vi "Manual Assembly DB_Nov2024.vi"() -> ()   [LabVIEW 2021]
uses:
  Classes/Assembly/Assembly Run.lvclass
  Classes/Workspace/Fixture Enum.ctl
  Classes/Workspace/Fixture.lvclass
  Classes/Controller/Controller.lvclass
  Classes/Assembly/Database Entry/Database Entry.lvclass
  SubVIs/component_tray_region.vi
  SubVIs/assembly_tray_region.vi
  SubVIs/PUT_region.vi
  <vilib>/JDP Science/JDP Science Common Utilities/JDP Utility.lvlib
  <vilib>/Utility/file.llb/Read Delimited Spreadsheet (string).vi
  Classes/Routine/Routine Enum.ctl
  Classes/Routine/Routine.lvclass
panel:
  out "Feet check":bool
  in  "Pick and Place 3":bool
  in  "Pick and Place 2":bool
  out "Assembly Type":string[](array[string])
  out "Assembly tray region":dbl
  out "Component tray region":dbl
  out "PUT Region":dbl
  in  "Clear All":bool
  in  "Assemble":bool
  in  "Pick and Place":bool
  in  "Dispense glue":bool
  in  "Go":bool
  in  "Routine":T1=enum."Dispense Epoxy"
  in  "Update":bool
  in  "Stage":i32(listbox)=-1
  in  "Stop":bool
  in  "Remove":bool
  in  "Add":bool
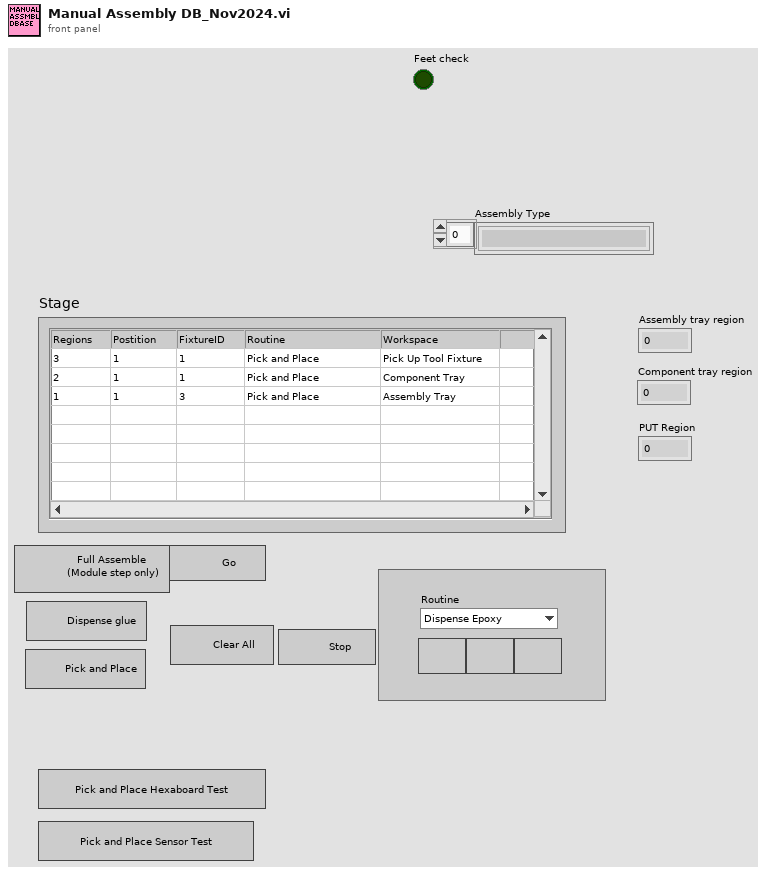
[diagram p1: front panel]
types:
  T1 = typedef "Routine.lvclass/Routine Enum.ctl" = enum16{"Primary Pick Up", "Secondary Pick Up", "Put Down All", "Secure Syringe", "Release Syringe", "Dispense Epoxy", "Pick Up All", "Put Down Secondary", "Full Assembly"}
  T2 = typedef "Fixture.lvclass/Fixture Enum.ctl" = enum16{"Assembly Tray", "Syringe Space", "Component", "Pick Up Tool", "Current Position"}
  T3 = typedef "File Paths.ctl" = cluster{"Glue Pattern Folder":path, "Carrier Tray Folder":path, "Pick Up Tool Fixture Folder":path, "Components Folder":path, "Bellows Tool Offset.txt":path, "Pick Up Tool Offset.txt":path, "Dispense Tip Offset.txt":path, "Log Files":path, "Gantry Assembly Map.txt":path, "Syringe and offset map.txt":path, "Controllers Folder":path, "Local dbase config":path}
  T4 = cluster{"Fixture ID":dbl, "Position":dbl, "Thickness":dbl}[]
  T5 = cluster{"Fixture ID":dbl, "Position":dbl, "Thickness":dbl}
  T6 = typedef "Controller.lvclass/Controllers.ctl" = cluster{"I-O.lvclass":refnum<class "I-O.lvclass">, "Gantry":refnum<k24>, "Dispenser":refnum<visa-resource-name>}
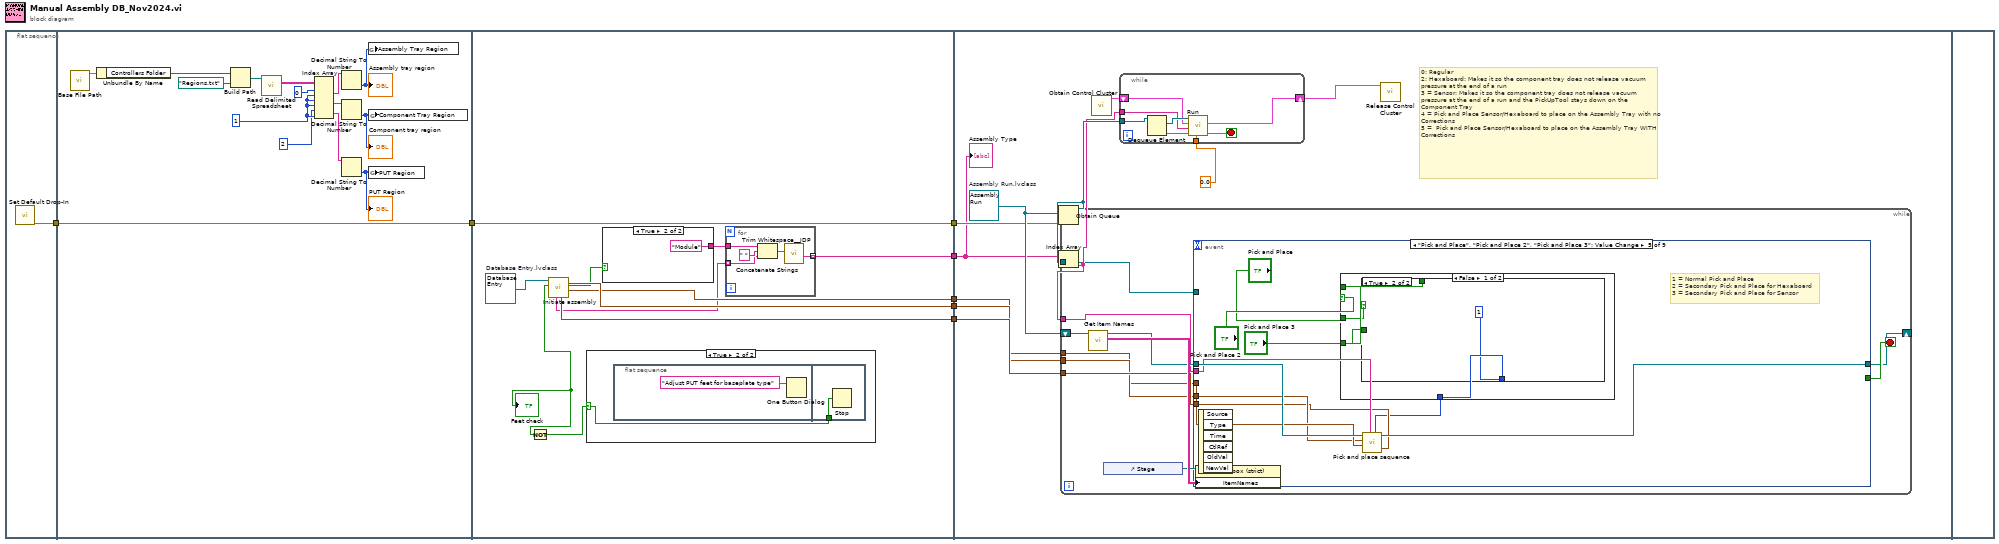
[diagram p0: block diagram]
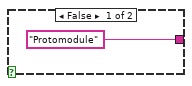
[diagram p3: hidden frame]
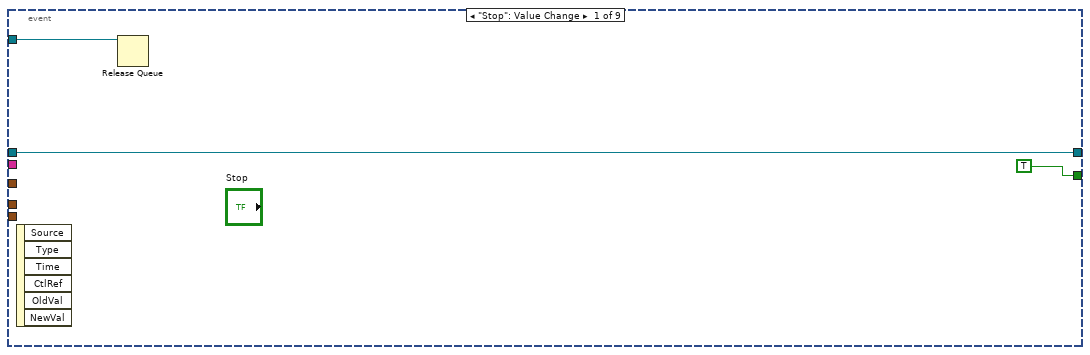
[diagram p4: hidden frame]
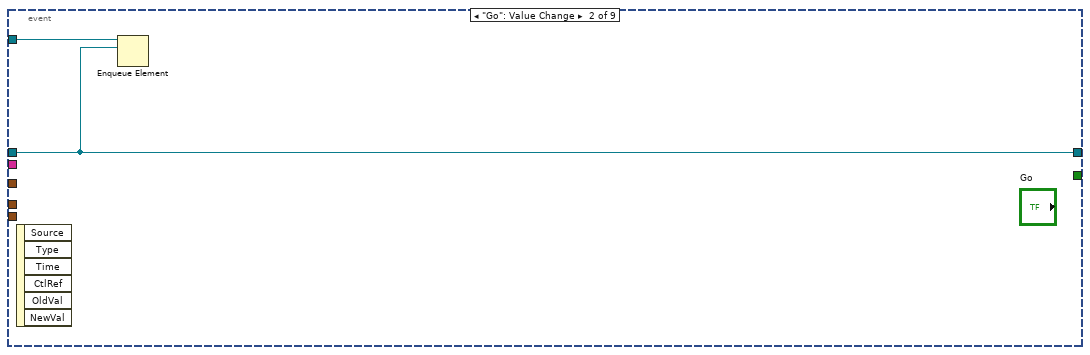
[diagram p5: hidden frame]
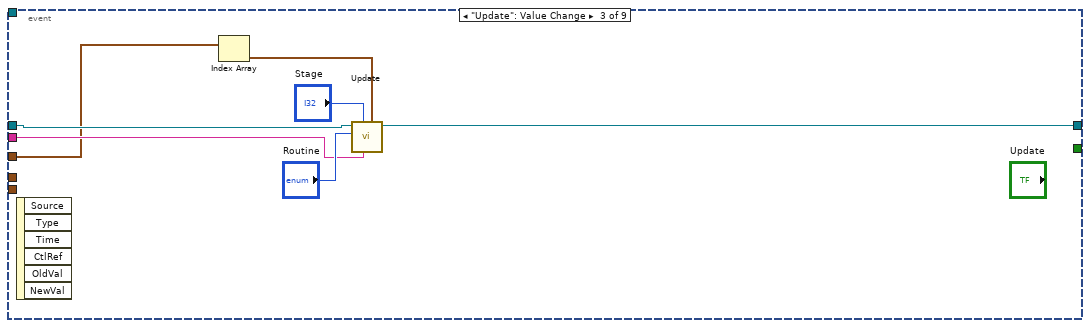
[diagram p6: hidden frame]
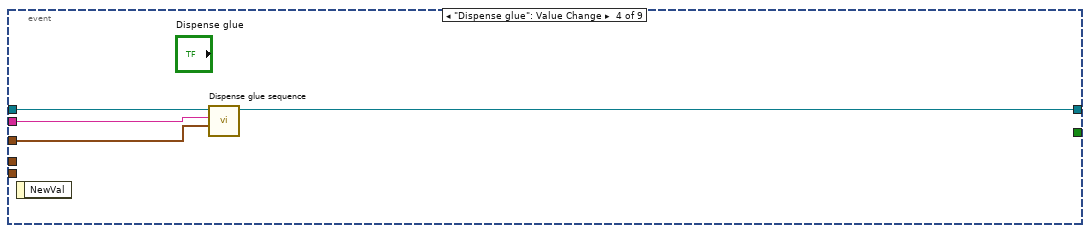
[diagram p7: hidden frame]
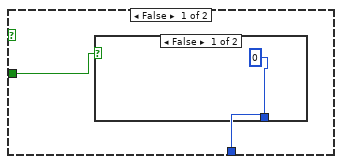
[diagram p8: hidden frame]
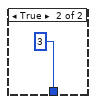
[diagram p9: hidden frame]
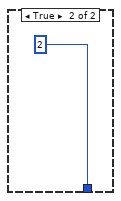
[diagram p10: hidden frame]
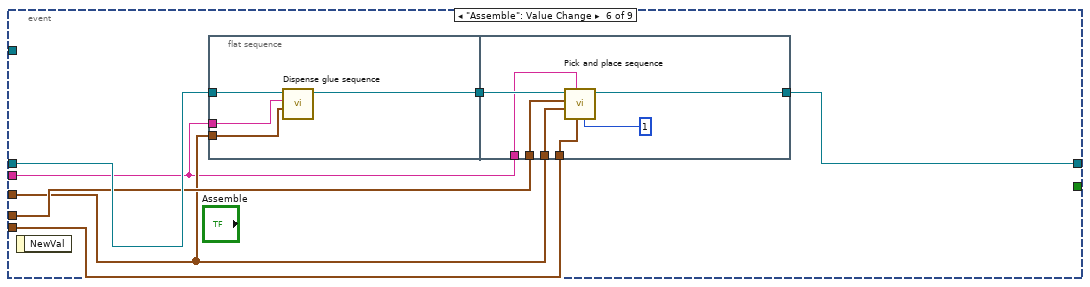
[diagram p11: hidden frame]
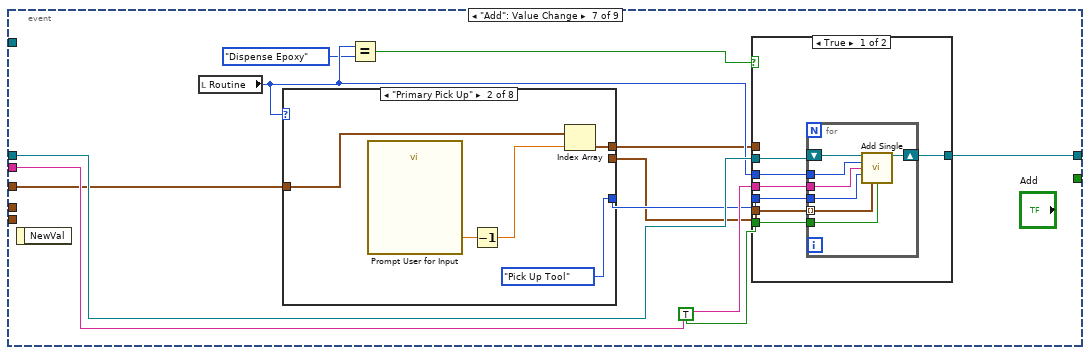
[diagram p12: hidden frame]
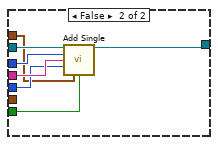
[diagram p13: hidden frame]
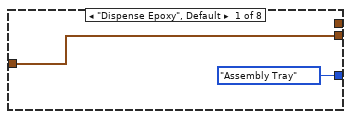
[diagram p14: hidden frame]
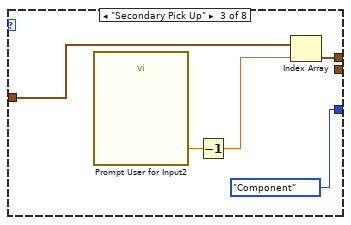
[diagram p15: hidden frame]
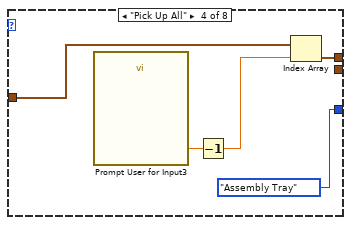
[diagram p16: hidden frame]
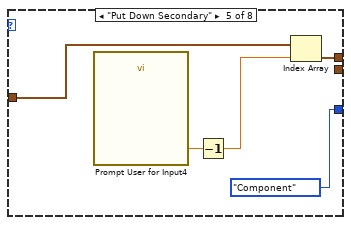
[diagram p17: hidden frame]
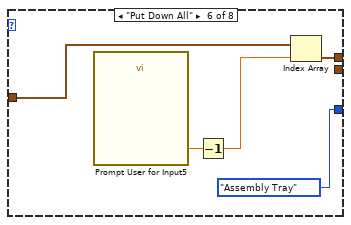
[diagram p18: hidden frame]
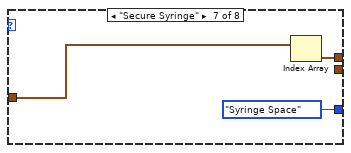
[diagram p19: hidden frame]
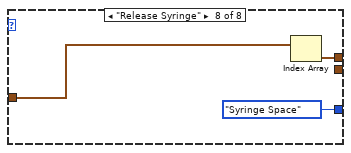
[diagram p20: hidden frame]
diagram:
  n1 = flat-sequence {
    tunnel: [w8] -> w5
    tunnel: [w9] -> w6
    tunnel: w5 -> [w9]
    tunnel: [w33] -> w7
    tunnel: w6 -> [w33]
    tunnel: [w32] -> w4
    tunnel: [w31] -> w3
    tunnel: [w30] -> w2
    tunnel: [w28] -> w1
    tunnel: w7 -> [w51]
    tunnel: w4 -> [w50]
    tunnel: w3 -> [w49]
    tunnel: w2 -> [w48]
    tunnel: w1 -> [w47]
    frame #0 {
      n2 = call "Set Default Drop-In.vi"() -> ("error out"=w8:errorcluster)  [unwired: 11 in]
    }
    frame #1 {
      w12 = 1 ("disabled index (col)")
      n3 = call "Base File Path.vi"() -> ("Paths Out"=w23:T3)  [unwired: 11 in]
      n4 = Unbundle By Name(w23) -> ("Controllers Folder"=w21:path)
      n5 = Build Path(base path=w21, name or relative path=path "Regions.txt") -> (appended path=w22:path)
      n6 = call-poly <vilib>:"Read Delimited Spreadsheet.vi"("file path (dialog if empty)"=w22) -> ("all rows"=w10:string[][])  [unwired: 9 in, 5 out]
      n7 = Index Array(array=w10, index (row) #1=0 ("index (row)"), index (col) #1=w12, index (row) #2=w12, index (col) #2=w12, index (row) #3=2 ("disabled index (row)"), index (col) #3=w12) -> (element #1=w15:string, element #2=w14:string, element #3=w16:string)
      n8 = Decimal String To Number(string=w15) -> (number=w18:i32)  [unwired: 2 in, 1 out]
      "Assembly tray region" <- w18
      n9 = Decimal String To Number(string=w14) -> (number=w19:i32)  [unwired: 2 in, 1 out]
      "Component tray region" <- w19
      n10 = Decimal String To Number(string=w16) -> (number=w17:i32)  [unwired: 2 in, 1 out]
      "PUT Region" <- w17
      n11 = global write "assembly_tray_region.vi" "Assembly Tray Region"(w18) -> ()
      n12 = global write "component_tray_region.vi" "Component Tray Region"(w19) -> ()
      n13 = global write "PUT_region.vi" "PUT Region"(w17) -> ()
    }
    frame #2 {
      w34 = refnum<class "Database Entry.lvclass"> refnum  # Database Entry.lvclass
      n14 = call "Initiate assembly.vi"("Database Entry in"=w34) -> ("Assembly Settings"=w30:T4, "Module?"=w27:bool, "Component Settings"=w32:T4, "PUT Settings"=w31:T4, "Assembly Type"=w25:string[], "Feet check"=w24:bool)  [unwired: 3 in, 2 out]
      "Feet check" <- w24
      n15 = Not(x=w24) -> (.not. x?=w26:bool)
      n16 = case shown="True" w26 {
        selector: w26 -> [_ w35]
        frame False {
        }
        frame True {
          n17 = flat-sequence {
            tunnel: w35 -> [w37]
            frame #0 {
              n18 = One Button Dialog(message="Adjust PUT feet for baseplate type") -> ()  [unwired: 1 in, 1 out]
            }
            frame #1 {
              n19 = Stop(stop? (T)=w37) -> ()
            }
          }
        }
      }
      n20 = case shown="True" w27 {
        tunnel: ["Protomodule" "Module"] -> w29
        frame False {
        }
        frame True {
        }
      }
      n21 = for {
        tunnel: w25 -> [w40] mode=indexing
        tunnel: w29 -> [w42]
        tunnel: [w38] -> w28 mode=indexing
        n22 = Concatenate Strings(w42, " " ("string"), w40) -> (w39:string)
        n23 = call <vilib>:"Trim Whitespace__JDP.vi"("String in"=w39) -> ("String out"=w38:string)  [unwired: 6 in]
      }
    }
    frame #3 {
      w53 = refnum<class "Assembly Run.lvclass"> refnum  # Assembly Run.lvclass
      # "0: Regular\n2: Hexaboard: Makes it so the component tray does not release vacuum pressure at the end of a run\n3 = Sensor: Makes it so the component tray does not release vacuum pressure at the end of a run and the PickUpTool stays down on the Component Tray\n4 = Pick and Place Sensor/Hexaboard to place on the Assembly Tray with no Corrections\n5 =  Pick and Place Sensor/Hexaboard to place on the Assembly Tray WITH Corrections"
      n24 = Obtain Queue(element data type=w53, error in (no error)=w51) -> (queue out=w55:refnum<queue>)  [unwired: 3 in, 2 out]
      n25 = Index Array(array=w47) -> (element=w46:string)  [unwired: 1 in]
      n26 = while {
        shift-right: [w60] -> _
        shift-left: w53 -> [w62]
        tunnel: w55 -> [w65]
        tunnel: w50 -> [w59]
        tunnel: w49 -> [w58]
        tunnel: w48 -> [w57]
        tunnel: w46 -> [w56]
        stop <- w66 stop-if-true
        n27 = call "Get Item Names.vi"("Assembly Run in"=w62) -> ("Item names"=w64:string[][], "Assembly Run out"=w61:refnum<class "Assembly Run.lvclass">)  [unwired: 8 in, 1 out]
        n28 = control-ref of="Stage"() -> (w63:refnum<vi>)
        n29 = event shown="[4] \"Pick and Place\", \"Pick and Place 2\", \"Pick and Place 3\": Value Change" {
          selector: _ -> [_ _ _ _ _ _ _ _ _]
          dyn-events: _ -> [_ _ _ _ _ _ _ _ _]
          timeout: _ -> [_ _ _ _ _ _ _ _ _]
          tunnel: [TRUE _ _ _ _ _ _ _ _] -> w66
          tunnel: w61 -> [w68 w70 w78 w82 w92 w109 w130 w188 _]
          tunnel: [w68 w70 w77 w81 w91 w108 w131 w187 w192] -> w60
          tunnel: w65 -> [w67 w71 _ _ _ _ _ _ w191]
          tunnel: w59 -> [_ _ _ _ w85 w105 _ _ _]
          tunnel: w58 -> [_ _ _ _ w86 w106 _ _ _]
          tunnel: w57 -> [_ _ w73 w80 w87 w104 w126 _ _]
          tunnel: w56 -> [_ _ w74 w79 w90 w103 w129 _ _]
          event "Stop": Value Change {
            n30 = event-data() -> ()  [unwired: 1 in, 6 out]
            n31 = Release Queue(queue=w67) -> ()  [unwired: 2 in, 3 out]
          }
          event "Go": Value Change {
            n32 = event-data() -> ()  [unwired: 1 in, 6 out]
            n33 = Enqueue Element(queue=w71, element=w70) -> ()  [unwired: 2 in, 3 out]
          }
          event "Update": Value Change {
            n34 = event-data() -> ()  [unwired: 1 in, 6 out]
            n35 = Index Array(array=w73) -> (element=w72:T5)  [unwired: 1 in]
            n36 = call "Update.vi"("Input Settings"=w72, "Assembly Type"=w74, "Row"="Stage", "Routine"="Routine", "Assembly Run in"=w78) -> ("Assembly Run out"=w77:refnum<class "Assembly Run.lvclass">)  [unwired: 5 in, 1 out]
          }
          event "Dispense glue": Value Change {
            n37 = event-data() -> ()  [unwired: 1 in, 1 out]
            n38 = call "Dispense glue sequence.vi"("Assembly Tray Settings Array"=w80, "Assembly Type"=w79, "Assembly Run in"=w82) -> ("Assembly Run out"=w81:refnum<class "Assembly Run.lvclass">)  [unwired: 7 in, 1 out]
          }
          event "Pick and Place", "Pick and Place 2", "Pick and Place 3": Value Change {
            # "1 = Normal Pick and Place\n2 = Secondary Pick and Place for Hexaboard\n3 = Secondary Pick and Place for Sensor"
            n39 = event-data() -> ()  [unwired: 1 in, 6 out]
            n40 = case shown="False" "Pick and Place 2" {
              tunnel: [w95 2] -> w84
              tunnel: "Pick and Place" -> [w96 _]
              tunnel: "Pick and Place 3" -> [w94 _]
              tunnel: "Pick and Place 3" -> [w93 _]
              frame False {
                n41 = case shown="True" w96 {
                  tunnel: [w98 1] -> w95
                  tunnel: w94 -> [_ _]
                  tunnel: w93 -> [w97 _]
                  frame False {
                    n42 = case shown="False" w97 {
                      tunnel: [0 3] -> w98
                      frame False {
                      }
                      frame True {
                      }
                    }
                  }
                  frame True {
                  }
                }
              }
              frame True {
              }
            }
            n43 = call "Pick and place sequence.vi"("Numeric"=w84, "Component Tray map"=w85, "Assembly Type"=w90, "Assembly Tray map"=w87, "PUT map"=w86, "Assembly Run in"=w92) -> ("Assembly Run out"=w91:refnum<class "Assembly Run.lvclass">)  [unwired: 4 in, 1 out]
          }
          event "Assemble": Value Change {
            n44 = event-data() -> ()  [unwired: 1 in, 1 out]
            n45 = flat-sequence {
              tunnel: [w112] -> w107
              tunnel: w109 -> [w113]
              tunnel: w104 -> [w111]
              tunnel: w103 -> [w110]
              tunnel: [w119] -> w108
              tunnel: w107 -> [w120]
              tunnel: w104 -> [w118]
              tunnel: w106 -> [w117]
              tunnel: w105 -> [w116]
              tunnel: w103 -> [w115]
              frame #0 {
                n46 = call "Dispense glue sequence.vi"("Assembly Tray Settings Array"=w111, "Assembly Type"=w110, "Assembly Run in"=w113) -> ("Assembly Run out"=w112:refnum<class "Assembly Run.lvclass">)  [unwired: 7 in, 1 out]
              }
              frame #1 {
                n47 = call "Pick and place sequence.vi"("Numeric"=1, "Component Tray map"=w116, "Assembly Type"=w115, "Assembly Tray map"=w118, "PUT map"=w117, "Assembly Run in"=w120) -> ("Assembly Run out"=w119:refnum<class "Assembly Run.lvclass">)  [unwired: 4 in, 1 out]
              }
            }
          }
          event "Add": Value Change {
            n48 = event-data() -> ()  [unwired: 1 in, 1 out]
            n49 = local read "Routine"() -> (w124:T1)
            n50 = case shown="\"Primary Pick Up\"" w124 {
              tunnel: [Fixture_Enum."Assembly Tray" ("Fixture") Fixture_Enum."Pick Up Tool" ("Fixture") Fixture_Enum."Component" ("Fixture") Fixture_Enum."Assembly Tray" ("Fixture") Fixture_Enum."Component" ("Fixture") Fixture_Enum."Assembly Tray" ("Fixture") Fixture_Enum."Syringe Space" ("Fixture") Fixture_Enum."Syringe Space" ("Fixture")] -> w128
              tunnel: w126 -> [w153 w158 w161 w166 w171 w175 w181 w184]
              tunnel: [_ w155 w160 w165 w170 w176 w180 w183] -> w121
              tunnel: [w153 _ _ _ _ _ _ _] -> w122
              frame "Dispense Epoxy", Default {
              }
              frame "Primary Pick Up" {
                n51 = call "Prompt User for Input"() -> ("Position"=w157:dbl)  [unwired: 17 in, 2 out]
                n52 = Decrement(x=w157) -> (x-1=w156:dbl)
                n53 = Index Array(array=w158, index=w156) -> (element=w155:T5)
              }
              frame "Secondary Pick Up" {
                n54 = call "Prompt User for Input2"() -> ("Position"=w163:dbl)  [unwired: 17 in, 2 out]
                n55 = Decrement(x=w163) -> (x-1=w162:dbl)
                n56 = Index Array(array=w161, index=w162) -> (element=w160:T5)
              }
              frame "Pick Up All" {
                n57 = call "Prompt User for Input3"() -> ("Position"=w168:dbl)  [unwired: 17 in, 2 out]
                n58 = Decrement(x=w168) -> (x-1=w167:dbl)
                n59 = Index Array(array=w166, index=w167) -> (element=w165:T5)
              }
              frame "Put Down Secondary" {
                n60 = call "Prompt User for Input4"() -> ("Position"=w173:dbl)  [unwired: 17 in, 2 out]
                n61 = Decrement(x=w173) -> (x-1=w172:dbl)
                n62 = Index Array(array=w171, index=w172) -> (element=w170:T5)
              }
              frame "Put Down All" {
                n63 = call "Prompt User for Input5"() -> ("Position"=w178:dbl)  [unwired: 17 in, 2 out]
                n64 = Decrement(x=w178) -> (x-1=w177:dbl)
                n65 = Index Array(array=w175, index=w177) -> (element=w176:T5)
              }
              frame "Secure Syringe" {
                n66 = Index Array(array=w181) -> (element=w180:T5)  [unwired: 1 in]
              }
              frame "Release Syringe" {
                n67 = Index Array(array=w184) -> (element=w183:T5)  [unwired: 1 in]
              }
            }
            n68 = Equal?(x=w124, y=Routine_Enum."Dispense Epoxy") -> (x = y?=w125:bool)
            n69 = case shown="True" w125 {
              tunnel: [w138 w152] -> w131
              tunnel: w130 -> [w137 w151]
              tunnel: w129 -> [w136 w150]
              tunnel: w128 -> [w135 w149]
              tunnel: w124 -> [w134 w148]
              tunnel: TRUE ("Auto") -> [w133 w147]
              tunnel: w122 -> [w132 _]
              tunnel: w121 -> [_ w146]
              frame True {
                n70 = for {
                  tunnel: w136 -> [w143]
                  tunnel: w135 -> [w142]
                  tunnel: w134 -> [w141]
                  tunnel: w133 -> [w140]
                  shift-right: [w145] -> w138
                  shift-left: w137 -> [w144]
                  tunnel: w132 -> [w139] mode=indexing
                  n71 = call-dynamic "Add Single.vi"("UI in"=w144, "Routine"=w141, "Assembly Type"=w143, "Fixture"=w142, "Input Settings"=w139, "Auto"=w140) -> ("UI out"=w145:refnum<class "Assembly Run.lvclass">)  [unwired: 8 in, 1 out]
                }
              }
              frame False {
                n72 = call-dynamic "Add Single.vi"("UI in"=w151, "Routine"=w148, "Assembly Type"=w150, "Fixture"=w149, "Input Settings"=w146, "Auto"=w147) -> ("UI out"=w152:refnum<class "Assembly Run.lvclass">)  [unwired: 8 in, 1 out]
              }
            }
          }
          event "Remove": Value Change {
            n73 = event-data() -> ()  [unwired: 1 in, 6 out]
            n74 = local read "Stage"() -> (w186:i32)
            n75 = call "Delete.vi"("Index"=w186, "Assembly In"=w188) -> ("Assembly Out"=w187:refnum<class "Assembly Run.lvclass">)  [unwired: 8 in, 1 out]
          }
          event "Clear All": Value Change {
            w192 = refnum<class "Assembly Run.lvclass"> refnum  # Assembly Run.lvclass
            n76 = event-data() -> ()  [unwired: 1 in, 6 out]
            n77 = Flush Queue(queue=w191) -> ()  [unwired: 1 in, 3 out]
            n78 = invoke on="Stage" class="MCListbox (strict)" method="Reinit To Default"() -> ()  [unwired: 3 in, 3 out]
            n79 = Build Array(FALSE) -> (w190:bool[])
            n80 = Array To Cluster(array=w190) -> ()  [unwired: 1 out]
          }
        }
        n81 = property class="MCListbox (strict)"(reference=w63, "ItemNames"=w64) -> ()  [unwired: 1 in, 2 out]
      }
      n82 = call "Obtain Control Cluster.vi"() -> ("Control Out"=w52:T6)  [unwired: 11 in]
      n83 = while {
        tunnel: w55 -> [w200]
        shift-right: [w195] -> w54
        shift-left: w52 -> [w196]
        tunnel: w46 -> [w194]
        tunnel: 0.0 -> [w193]
        stop <- w197 stop-if-true
        n84 = Dequeue Element(queue=w200) -> (element=w199:refnum<class "Assembly Run.lvclass">, error out=w198:errorcluster)  [unwired: 2 in, 2 out]
        n85 = call-dynamic "Run.vi"("Pickup_Test_Number"=w193, "error in (no error)"=w198, "Assembly Type"=w194, "Control In"=w196, "Assembly In"=w199) -> ("error out"=w197:errorcluster, "Control Out"=w195:T6)  [unwired: 4 in, 1 out]
      }
      n86 = call "Release Control Cluster.vi"("output cluster"=w54) -> ()  [unwired: 11 in]
      "Assembly Type" <- w47
    }
    frame #4 {
    }
  }
